vi "get_display_voltage_current_and_mode.vi"(8 "error in":errorcluster, 11 "VISA resource name":refnum<visa-resource-name>="COM1") -> (0 "error out":errorcluster, 3 "VISA resource name out":refnum<visa-resource-name>)   [LabVIEW 2020]
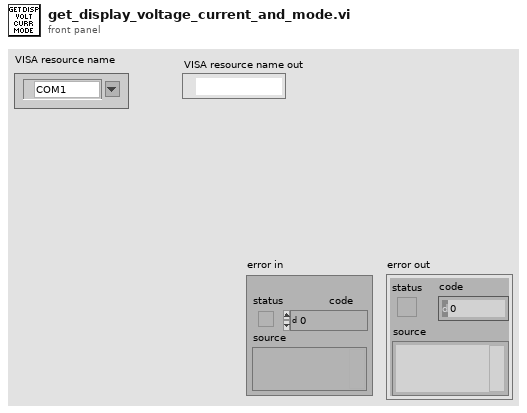
[diagram p1: front panel]
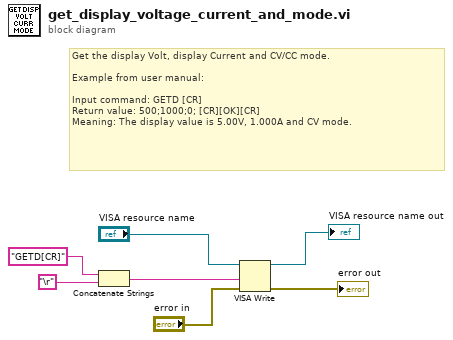
[diagram p0: block diagram]
diagram:
  # "Get the display Volt, display Current and CV/CC mode.\n\nExample from user manual:\n\nInput command: GETD [CR]\nReturn value: 500;1000;0; [CR][OK][CR]\nMeaning: The display value is 5.00V, 1.000A and CV mode."
  n1 = Concatenate Strings("GETD[CR]" ("Command"), "\r") -> (w4:string)
  n2 = VISA Write(VISA resource name="VISA resource name", write buffer=w4, error in (no error)="error in") -> (VISA resource name out=→"VISA resource name out":refnum<visa-resource-name>, error out=→"error out":errorcluster)  [unwired: 1 out]
